vi "1. Used as parameters parsed by CSM.vi"() -> ()   [LabVIEW 2017]
uses:
  INI-Static-Variable-Support/INI-Static-Variable-Support.lvlib
panel:
  out "State Queue":string
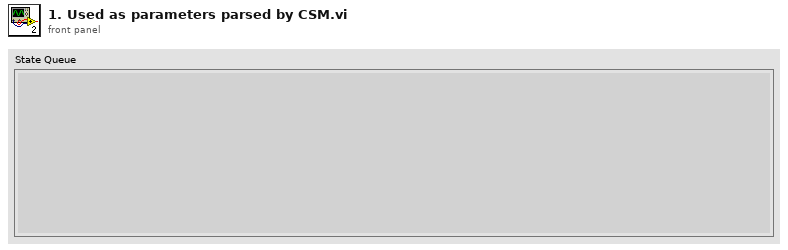
[diagram p1: front panel]
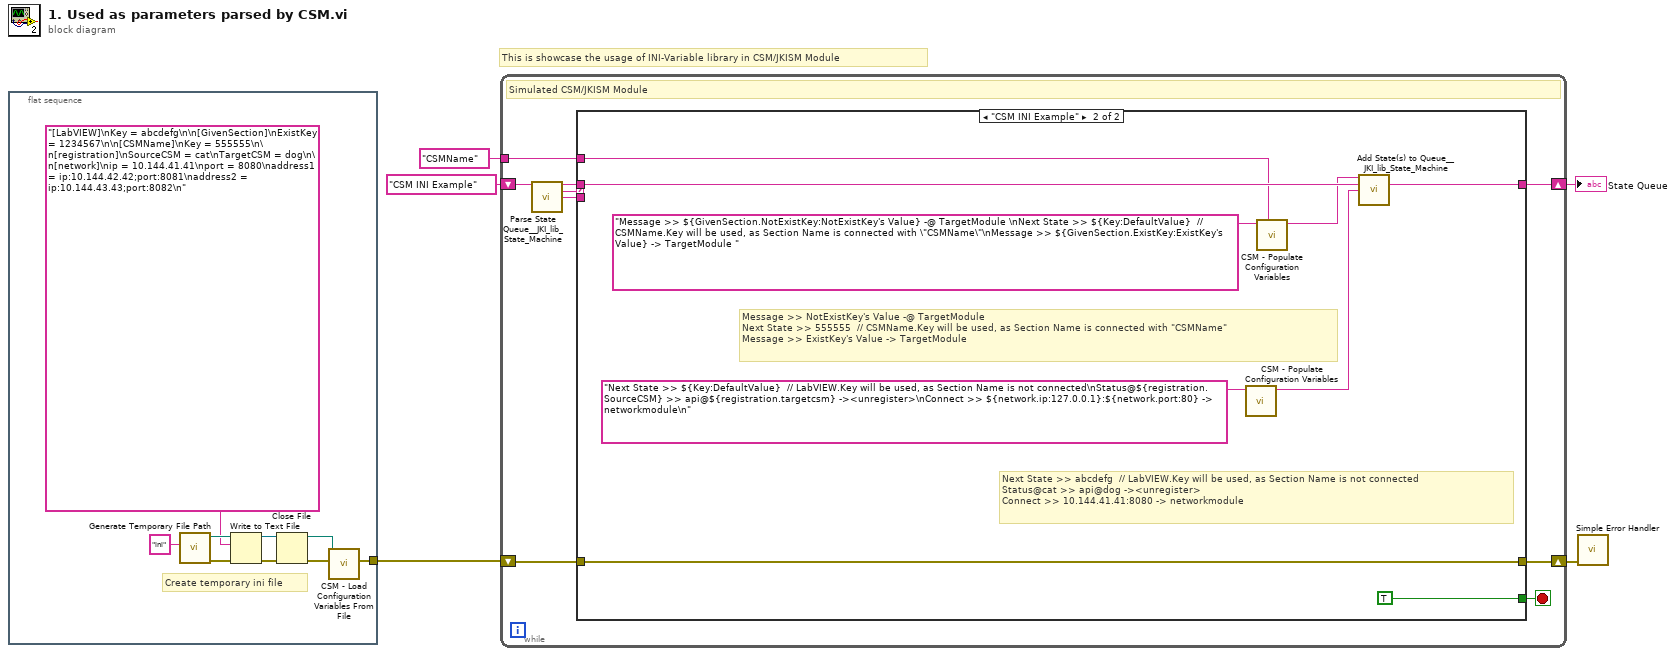
[diagram p0: block diagram]
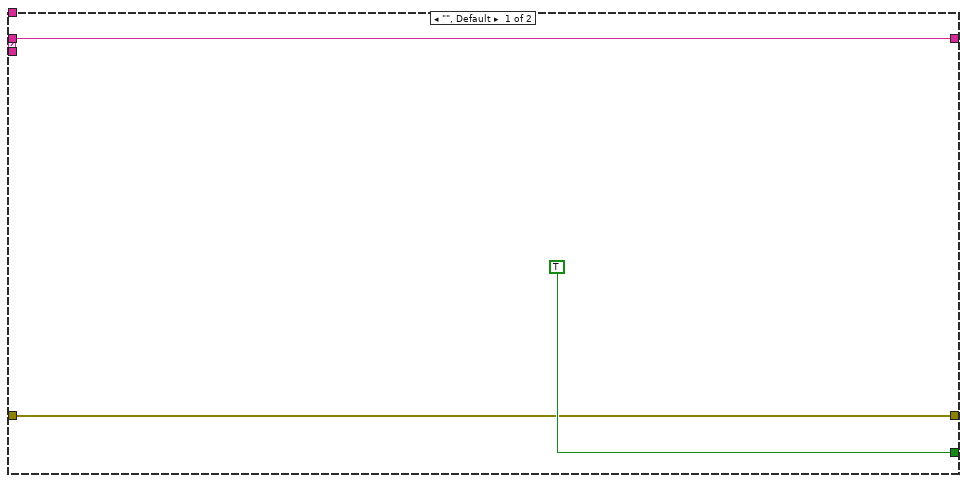
[diagram p2: hidden frame]
diagram:
  # "This is showcase the usage of INI-Variable library in CSM/JKISM Module"
  n1 = flat-sequence {
    tunnel: [w8] -> w2
    frame #0 {
      # "Create temporary ini file"
      n2 = call <vilib>:"Generate Temporary File Path.vi"("Temporary File Extension (tmp)"="ini") -> ("error out"=w14:errorcluster, "Unique Temporary File Path"=w11:path)  [unwired: 9 in]
      n3 = Write to Text File(file (use dialog)=w11, text="[LabVIEW]\nKey = abcdefg\n\n[GivenSection]\nExistKey = 1234567\n\n[CSMName]\nKey = 555555\n\n[registration]\nSourceCSM = cat\nTargetCSM = dog\n\n[network]\nip = 10.144.41.41\nport = 8080\naddress1 = ip:10.144.42.42;port:8081\naddress2 = ip:10.144.43.43;port:8082\n", error in=w14) -> (refnum out=w10:refnum<file>, error out=w12:errorcluster)  [unwired: 1 in, 1 out]
      n4 = Close File(refnum=w10, error in=w12) -> (path=w6:path, error out=w9:errorcluster)
      n5 = call "CSM - Load Configuration Variables From File.vi"("error in (no error)"=w9, "Path"=w6) -> ("error out"=w8:errorcluster)  [unwired: 7 in]
    }
  }
  n6 = while "Communicable State Machine(CSM) 2025" {
    shift-right: [w21] -> w4
    shift-left: "CSM INI Example" ("State Queue") -> [w23]
    shift-right: [w16] -> w1
    shift-left: w2 -> [w17]
    tunnel: "CSMName" ("State Queue") -> [w15]
    stop <- w18 stop-if-true
    # "Simulated CSM/JKISM Module"
    n7 = call <vilib>:"Parse State Queue__JKI_lib_State_Machine.vi"("State Queue"=w23) -> ("Remaining States"=w22:string, "Current State"=w20:string, "Arguments"=w19:string)  [unwired: 12 in]
    n8 = case shown="\"CSM INI Example\"" w20 {
      tunnel: w22 -> [w26 w33]
      tunnel: [w26 w32] -> w21
      tunnel: w19 -> [_ _]
      tunnel: [TRUE TRUE] -> w18
      tunnel: w17 -> [w24 w34]
      tunnel: [w24 w34] -> w16
      tunnel: w15 -> [_ w29]
      frame "", Default {
      }
      frame "CSM INI Example" {
        # "Message >> NotExistKey's Value -@ TargetModule \nNext State >> 555555  // CSMName.Key will be used, as Section Name is connected with \"CSMName\"\nMessage >> ExistKey's Value -> TargetModule"
        # "Next State >> abcdefg  // LabVIEW.Key will be used, as Section Name is not connected\nStatus@cat >> api@dog -><unregister>\nConnect >> 10.144.41.41:8080 -> networkmodule"
        n9 = call "CSM - Populate Configuration Variables.vi"("String in"="Next State >> ${Key:DefaultValue}  // LabVIEW.Key will be used, as Section Name is not connected\nStatus@${registration.SourceCSM} >> api@${registration.targetcsm} -><unregister>\nConnect >> ${network.ip:127.0.0.1}:${network.port:80} -> networkmodule\n") -> ("String out"=w27:string)  [unwired: 7 in, 1 out]
        n10 = call "CSM - Populate Configuration Variables.vi"("Section Name(\"\" as Default)"=w29, "String in"="Message >> ${GivenSection.NotExistKey:NotExistKey's Value} -@ TargetModule \nNext State >> ${Key:DefaultValue}  // CSMName.Key will be used, as Section Name is connected with \"CSMName\"\nMessage >> ${GivenSection.ExistKey:ExistKey's Value} -> TargetModule ") -> ("String out"=w31:string)  [unwired: 6 in, 1 out]
        n11 = call <vilib>:"Add State(s) to Queue__JKI_lib_State_Machine.vi"("State(s) in Front (\"\")"=w31, "State(s) in (\"\")"=w33, "State(s) at Back (\"\")"=w27) -> ("States Out"=w32:string)  [unwired: 12 in]
      }
    }
  }
  "State Queue" <- w4
  n12 = call <vilib>:"Simple Error Handler.vi"("error in (no error)"=w1) -> ()  [unwired: 4 in, 5 out]
